vi "art联动采集V4.0.vi"() -> ()   [LabVIEW 2016]
uses:
  <vilib>/Instr/_visa.llb/VISA Configure Serial Port (Instr).vi
  <vilib>/Utility/file.llb/Write Delimited Spreadsheet (DBL).vi
panel:
  in  "定位模式":bool
  in  "X终点":dbl
  in  "Y终点":dbl
  in  "高级设置":bool
  in  "Y轴回零速度":dbl=15000.0
  in  "X轴回零速度":dbl=15000.0
  in  "细分设置":dbl=8.0
  in  "等待时间":u32=40
  in  "文件保存":path=path "D:/" caption="保存路径"
  out "行用时（s）":dbl
  out "time（行）":u32
  out "hDevice out":i32=253955776
  out "error out":errorcluster caption="错误输出"
  in  "退出扫描(Esc)":bool
  out "N_Length":i32=16384
  out "M_Length":i32
  out "hDevice":i32=241832032
  out "pulDDR2Length":u32=256
  out "总用时（s）":dbl
  out "毫秒计时值":u32=3586537
  out "数组":dbl[][](array[numeric])=[[58819.77200735986, 88200.32943600747]]
  out "强度图":dbl[][](graph)=[[58819.77200735986, 88200.32943600747]]
  out "judge":dbl
  out "Xloop":dbl
  out "幅频谱":dbl[](graph)
  out "时域谱":dbl[](graph)
  out "错误输出":errorcluster
  in  "启动":bool
  in  "开始扫描":bool
  in  "X归零":bool
  in  "Y归零":bool
  in  "Y起点":dbl
  in  "Y轴速度":dbl=9000.0
  in  "X轴速度":dbl=9000.0
  out "电机状态":bool
  in  "电机端口":refnum<visa-resource-name>="COM6"
  out "Yloop":dbl=1.0
  out "X扫描范围":dbl=150.0
  out "Y扫描范围":dbl=75.0
  out "Y序":i32
  in  "X起点":dbl
  out "Y(mm)":dbl
  out "x+y 2":dbl=3.0
  in  "Y步进":dbl=1.0
  in  "精度":dbl=0.001
  in  "电机急停":bool
  out "X（mm）":dbl
  out "x+y":dbl=1.0
  in  "X步进":dbl=1.0
  # "实时坐标"
  # "时域谱"
  # "频域谱"
  # "扫描参数"
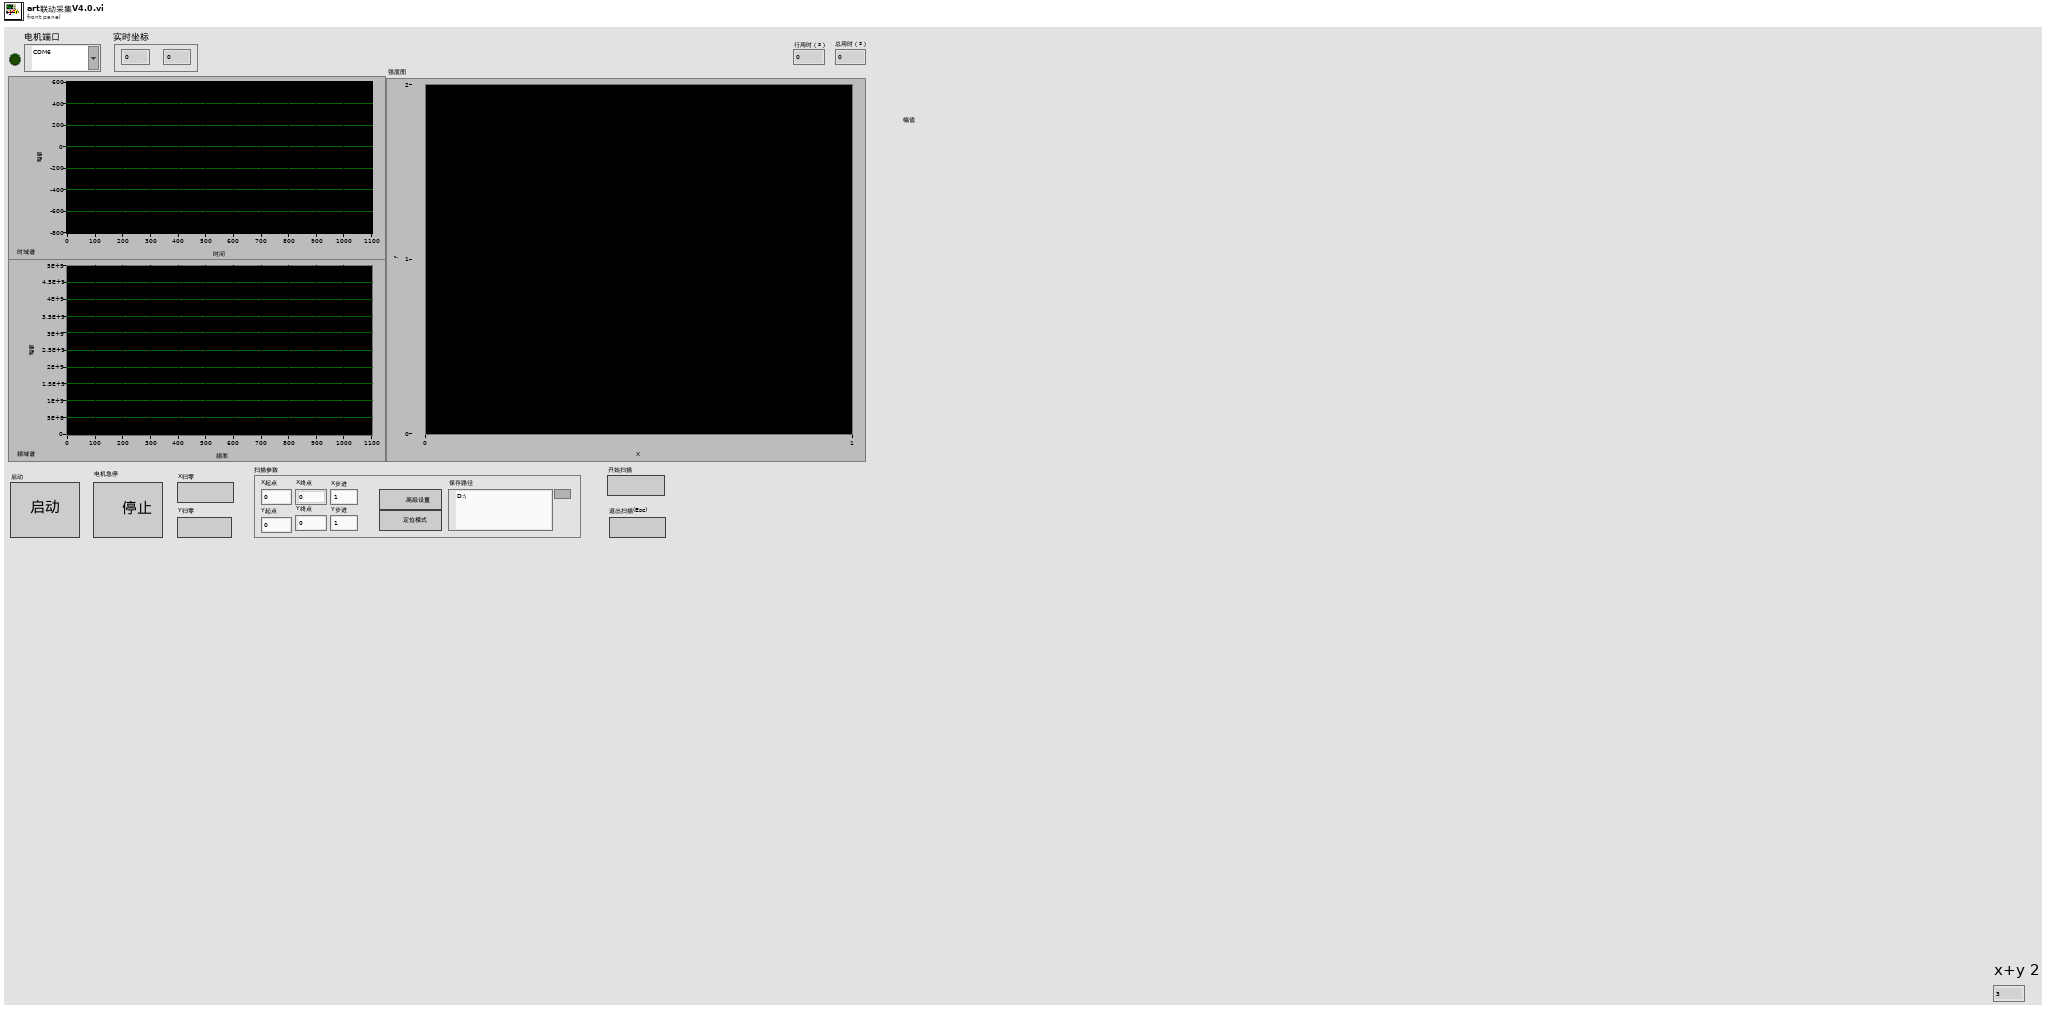
[diagram p1: front panel]
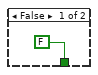
[diagram p2: hidden frame]
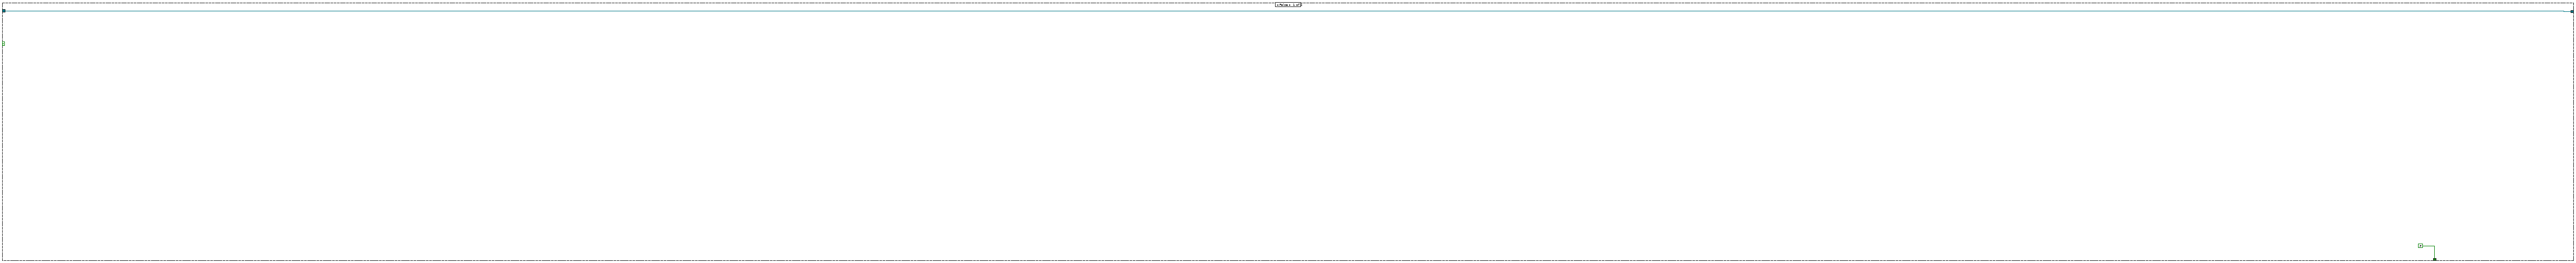
[diagram p3: hidden frame]
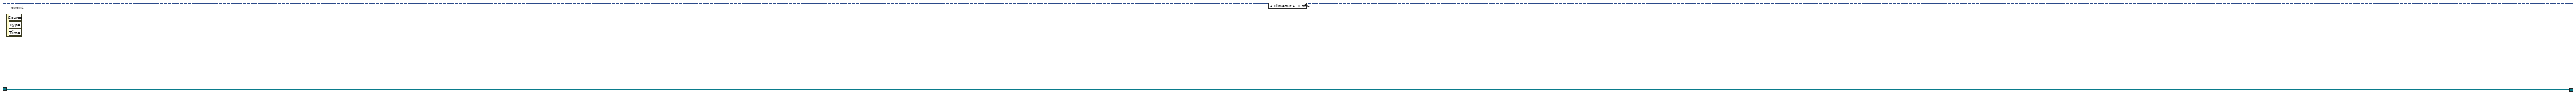
[diagram p4: hidden frame]
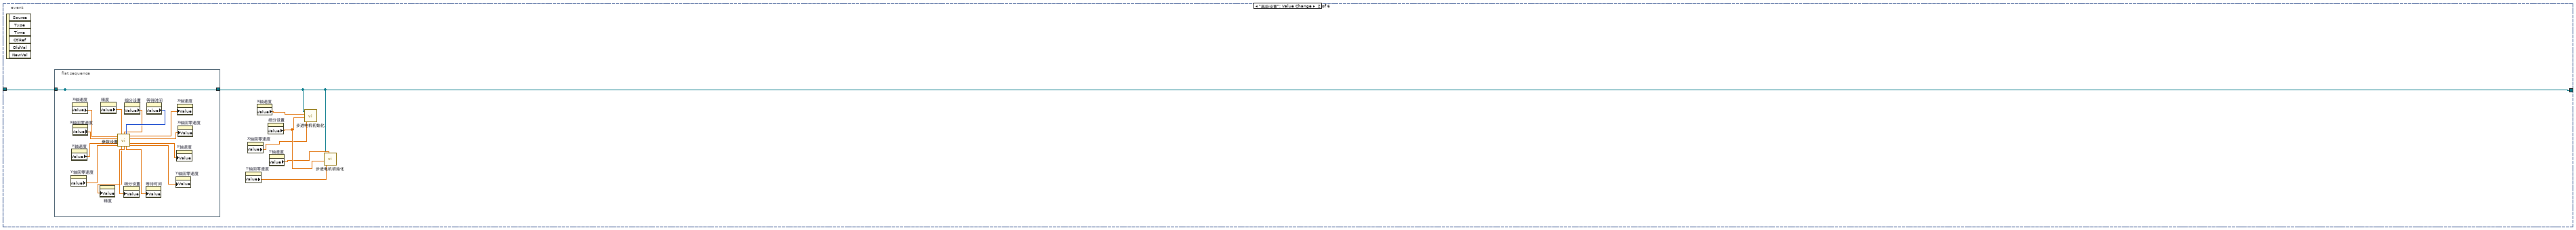
[diagram p5: hidden frame]
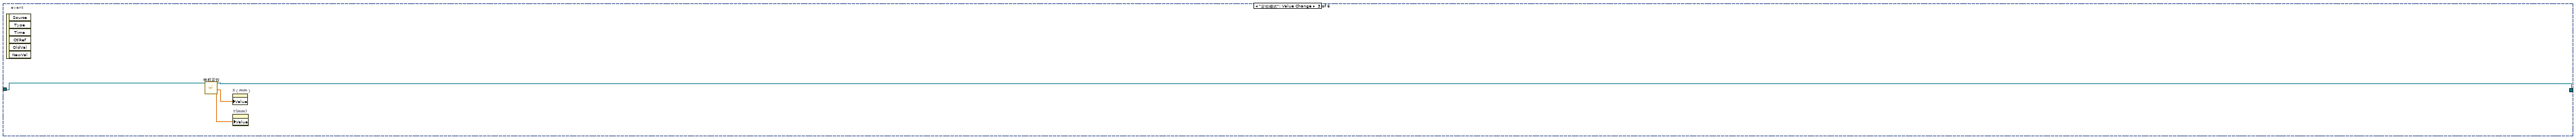
[diagram p6: hidden frame]
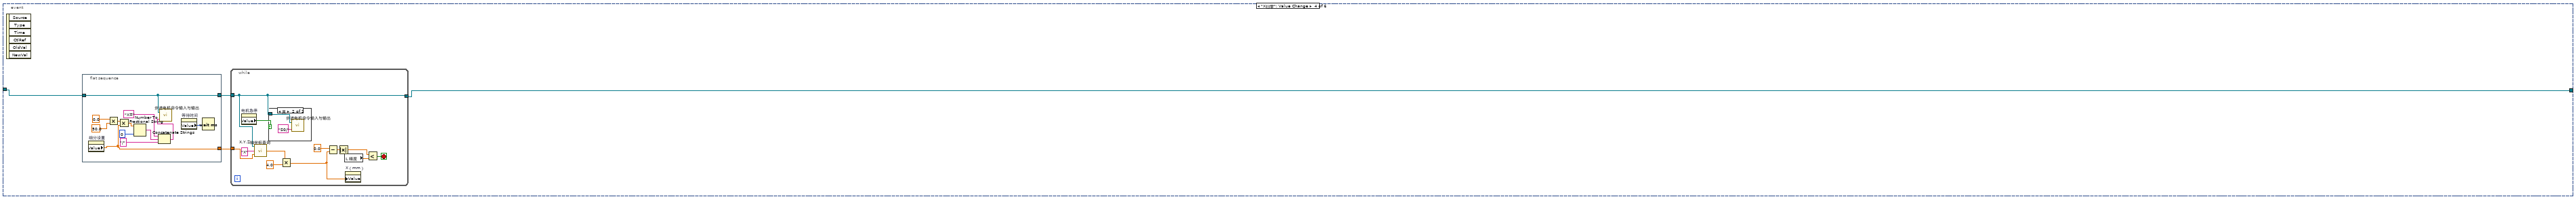
[diagram p7: hidden frame]
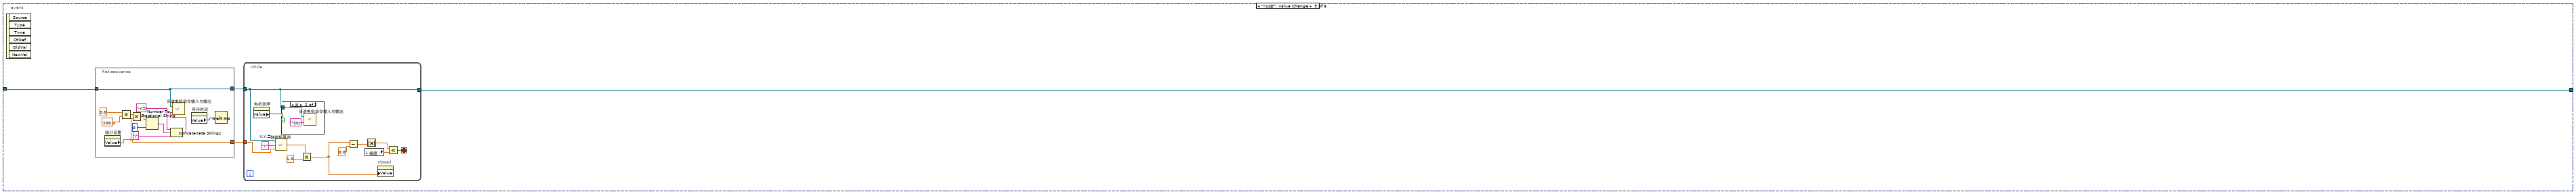
[diagram p9: hidden frame]
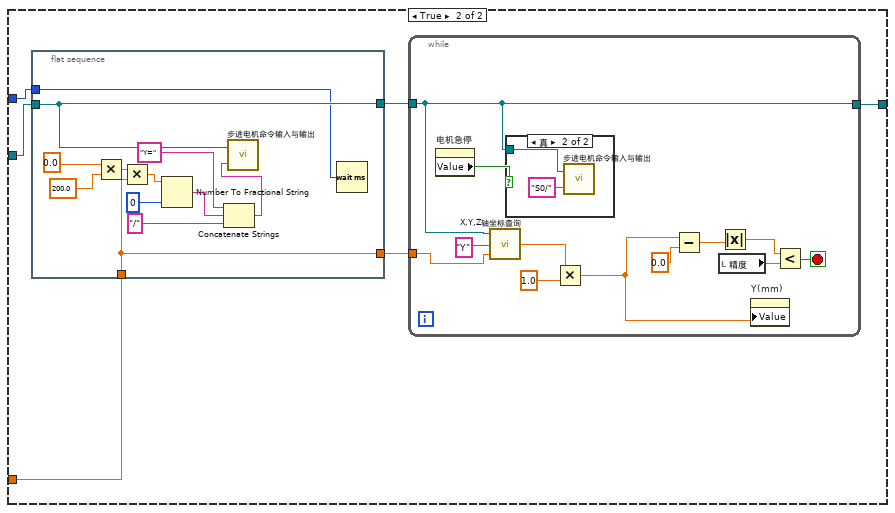
[diagram p15: hidden frame]
diagram:
  n1 = while {
    stop <- w1 stop-if-true
    n2 = case shown="真" "启动" {
      tunnel: [FALSE ("ESC") w8] -> w1
      frame False {
      }
      frame True {
        w23 = 0  # OutClockSource
        w24 = 0  # bClockSourceDir
        w26 = 10000000  # Frequency
        w27 = 0  # ClockSource
        w28 = 0  # TrigLevelVolt
        w15 = 1
        w29 = 0  # TriggerDir
        w30 = 0  # TriggerSource
        w31 = 0  # ATRTriggerChannel
        w32 = 0  # TriggerMode
        w16 = 4096  # N_Length
        w17 = 0  # M_Length
        w33 = 1  # CouplingType
        w34 = 0  # DeviceLgcID
        w44 = u16 0 items=["无", "XON/XOFF", "RTS/CTS", "XON/XOFF & RTS/CTS", "DTR/DSR", "XON/XOFF & DTR/DSR"] ("flow control (0:none)")
        w45 = u16 10 items=["1.0"=10, "1.5"=15, "2.0"=20] ("stop bits (10: 1 bit)")
        # "3"
        # "2"
        # "1"
        n3 = call-poly "VISA Configure Serial Port"("VISA resource name"="电机端口", "baud rate (9600)"=u32 9600, "data bits (8)"=u16 8, "parity (0:none)"=enum16{"None", "Odd", "Even", "Mark", "Space"}."None", "stop bits (10: 1 bit)"=w45, "flow control (0:none)"=w44) -> ("VISA resource name out"=w36:refnum<visa-resource-name>, "error out"=→"error out":errorcluster)  [unwired: 1 in, 7 out]
        n4 = Build Array "InputRange"(w15, w15, w15, w15) -> (w14:i32[])
        n5 = dll-call lib="PTH2aabs CUsersH301Desktopart闭环扫描程序采集卡控制INFamd64PCI8502_32.dll" fn="PCI8502_CreateDevice" label="CreateDevice"("DeviceLgcID"=w34) -> (w21:i32)  [unwired: 4 in, 2 out]
        n6 = property on="细分设置" class="DigNum (严格)"() -> ("Value"=w7:dbl)  [unwired: 2 in, 2 out]
        n7 = Build Array (concatenate) "InitDeviceAD"(w26, w14, w33, w17, w16, w32, w31, w30, w29, w28, w27, w24, w23) -> (w25:i32[])
        n8 = call "步进电机初始化.vi"("回零速度"="X轴回零速度", "细分设置"=w7, "X轴速度"="X轴速度", "串口通信端口"=w36) -> ()  [unwired: 2 in, 1 out]
        n9 = dll-call lib="PTH2aabs CUsersH301Desktopart闭环扫描程序采集卡控制INFamd64PCI8502_32.dll" fn="PCI8502_GetDDR2Length" label="GetDDR2Length"("hDevice"=w21, "pulDDR2Length"=u32 0) -> ("hDevice"=w20:i32, "pulDDR2Length"=→"pulDDR2Length":u32)  [unwired: 4 in, 2 out]
        n10 = call "步进电机初始化.vi"("Y轴速度"="Y轴速度", "回零速度"="Y轴回零速度", "细分设置"=w7, "串口通信端口"=w36) -> ()  [unwired: 2 in, 1 out]
        n11 = call "步进电机命令输入与输出.vi"("输入字符串"="?R/", "串口通信端口"=w36) -> ("返回字符串"=w41:string)
        n12 = dll-call lib="PTH2aabs CUsersH301Desktopart闭环扫描程序采集卡控制INFamd64PCI8502_32.dll" fn="PCI8502_InitDeviceAD" label="InitDeviceAD"("hDevice"=w20, "pADPara"=w25) -> ("hDevice"=→"hDevice":i32)  [unwired: 5 in, 2 out]
        n13 = String Subset(string=w41, offset (0)=0 ("偏移量(0)"), length (rest)=2 ("长度（剩余）")) -> (substring=w38:string)
        n14 = Equal?(x=w38, y="OK") -> (x = y?=w35:bool)
        "电机状态" <- w35
        n15 = case shown="真" w35 {
          tunnel: w36 -> [w51 w54]
          tunnel: [w51 w53] -> w9
          tunnel: [FALSE ("ESC") w52] -> w8
          frame False {
          }
          frame True {
            n16 = while {
              tunnel: w54 -> [w58]
              tunnel: [w57] -> w53
              tunnel: ["退出扫描(Esc)"] -> w52
              stop <- "退出扫描(Esc)" stop-if-true
              n17 = event shown="[5] \"开始扫描\": 值改变" {
                selector: _ -> [_ _ _ _ _ _]
                dyn-events: _ -> [_ _ _ _ _ _]
                timeout: 1 -> [_ _ _ _ _ _]
                tunnel: w58 -> [w59 w66 w85 w89 w119 w170]
                tunnel: [w59 w60 w84 w87 w117 w163] -> w57
                event Timeout {
                  n18 = event-data() -> ()  [unwired: 1 in, 3 out]
                }
                event "高级设置": Value Change {
                  n19 = event-data() -> ()  [unwired: 1 in, 6 out]
                  n20 = flat-sequence {
                    tunnel: w66 -> [w67]
                    tunnel: [w67] -> _
                    tunnel: [w67] -> w60
                    frame #0 {
                      n21 = property on="Y轴回零速度" class="DigNum (严格)"() -> ("Value"=w71:dbl)  [unwired: 2 in, 2 out]
                      n22 = property on="Y轴速度" class="DigNum (严格)"() -> ("Value"=w70:dbl)  [unwired: 2 in, 2 out]
                      n23 = property on="X轴速度" class="DigNum (严格)"() -> ("Value"=w68:dbl)  [unwired: 2 in, 2 out]
                      n24 = property on="X轴回零速度" class="DigNum (严格)"() -> ("Value"=w69:dbl)  [unwired: 2 in, 2 out]
                      n25 = property on="精度" class="DigNum (严格)"() -> ("Value"=w75:dbl)  [unwired: 2 in, 2 out]
                      n26 = property on="细分设置" class="DigNum (严格)"() -> ("Value"=w76:dbl)  [unwired: 2 in, 2 out]
                      n27 = property on="等待时间" class="DigNum (严格)"() -> ("Value"=w77:u32)  [unwired: 2 in, 2 out]
                      n28 = call "参数设置.vi"("X轴速度"=w68, "精度"=w75, "细分设置"=w76, "等待时间"=w77, "X轴回零速度"=w69, "Y轴速度"=w70, "Y轴回零速度"=w71) -> ("X轴速度"=w78:dbl, "X轴回零速度"=w79:dbl, "Y轴速度"=w80:dbl, "精度"=w72:dbl, "细分设置"=w73:dbl, "等待时间"=w74:dbl, "Y轴回零速度"=w81:dbl)  [unwired: 2 in]
                      n29 = property on="精度" class="DigNum (严格)"("Value"=w72) -> ()  [unwired: 2 in, 2 out]
                      n30 = property on="细分设置" class="DigNum (严格)"("Value"=w73) -> ()  [unwired: 2 in, 2 out]
                      n31 = property on="等待时间" class="DigNum (严格)"("Value"=w74) -> ()  [unwired: 2 in, 2 out]
                      n32 = property on="Y轴回零速度" class="DigNum (严格)"("Value"=w81) -> ()  [unwired: 2 in, 2 out]
                      n33 = property on="Y轴速度" class="DigNum (严格)"("Value"=w80) -> ()  [unwired: 2 in, 2 out]
                      n34 = property on="X轴速度" class="DigNum (严格)"("Value"=w78) -> ()  [unwired: 2 in, 2 out]
                      n35 = property on="X轴回零速度" class="DigNum (严格)"("Value"=w79) -> ()  [unwired: 2 in, 2 out]
                    }
                  }
                  n36 = property on="Y轴回零速度" class="DigNum (严格)"() -> ("Value"=w62:dbl)  [unwired: 2 in, 2 out]
                  n37 = property on="X轴回零速度" class="DigNum (严格)"() -> ("Value"=w63:dbl)  [unwired: 2 in, 2 out]
                  n38 = property on="X轴速度" class="DigNum (严格)"() -> ("Value"=w64:dbl)  [unwired: 2 in, 2 out]
                  n39 = property on="细分设置" class="DigNum (严格)"() -> ("Value"=w65:dbl)  [unwired: 2 in, 2 out]
                  n40 = property on="Y轴速度" class="DigNum (严格)"() -> ("Value"=w61:dbl)  [unwired: 2 in, 2 out]
                  n41 = call "步进电机初始化.vi"("回零速度"=w63, "细分设置"=w65, "X轴速度"=w64, "串口通信端口"=w60) -> ()  [unwired: 2 in, 1 out]
                  n42 = call "步进电机初始化.vi"("Y轴速度"=w61, "回零速度"=w62, "细分设置"=w65, "串口通信端口"=w60) -> ()  [unwired: 2 in, 1 out]
                }
                event "定位模式": Value Change {
                  n43 = event-data() -> ()  [unwired: 1 in, 6 out]
                  n44 = call "电机定位.vi"("VISA I"=w85) -> ("Y"=w82:dbl, "X"=w83:dbl, "VISA O"=w84:refnum<visa-resource-name>)  [unwired: 8 in]
                  n45 = property on="X（mm）" class="DigNum (严格)"("Value"=w83) -> ()  [unwired: 2 in, 2 out]
                  n46 = property on="Y(mm)" class="DigNum (严格)"("Value"=w82) -> ()  [unwired: 2 in, 2 out]
                }
                event "X归零": Value Change {
                  n47 = event-data() -> ()  [unwired: 1 in, 6 out]
                  n48 = flat-sequence {
                    tunnel: w89 -> [w93]
                    tunnel: [w93] -> w88
                    tunnel: [w90] -> w86
                    frame #0 {
                      n49 = property on="细分设置" class="DigNum (严格)"() -> ("Value"=w90:dbl)  [unwired: 2 in, 2 out]
                      n50 = Multiply(x=0.0, y=50.0) -> (x*y=w96:dbl)
                      n51 = Multiply(x=w96, y=w90) -> (x*y=w101:dbl)
                      n52 = Number To Fractional String(number=w101, precision (6)=i16 0 ("精度(6)")) -> (F-format string=w99:string)  [unwired: 2 out]
                      n53 = Concatenate Strings("X=" ("字符串"), w99, "/" ("字符串")) -> (w94:string)
                      n54 = call "步进电机命令输入与输出.vi"("输入字符串"=w94, "串口通信端口"=w93) -> ()  [unwired: 1 out]
                      n55 = property on="等待时间" class="DigNum (严格)"() -> ("Value"=w91:u32)  [unwired: 2 in, 2 out]
                      n56 = Wait (ms)(milliseconds to wait=w91) -> ()  [unwired: 1 out]
                    }
                  }
                  n57 = while {
                    tunnel: [w103] -> w87
                    tunnel: w88 -> [w103]
                    tunnel: w86 -> [w102]
                    stop <- w109 stop-if-true
                    n58 = property on="电机急停" class="Bool (严格)"() -> ("Value"=w110:bool)  [unwired: 2 in, 2 out]
                    n59 = call "X,Y,Z轴坐标查询.vi"("细分设置"=w102, "查询坐标轴"="X", "串口通信端口"=w103) -> ("坐标(mm)"=w111:dbl)
                    n60 = case shown="真" w110 {
                      tunnel: w103 -> [_ w114]
                      frame False {
                      }
                      frame True {
                        n61 = call "步进电机命令输入与输出.vi"("输入字符串"="S0/", "串口通信端口"=w114) -> ()  [unwired: 1 out]
                      }
                    }
                    n62 = Multiply(x=w111, y=4.0 ("x")) -> (x*y=w107:dbl)
                    n63 = Subtract(x=0.0, y=w107) -> (x-y=w106:dbl)
                    n64 = Absolute Value(x=w106) -> (abs(x)=w105:dbl)
                    n65 = local read "精度"() -> (w108:dbl)
                    n66 = property on="X（mm）" class="DigNum (严格)"("Value"=w107) -> ()  [unwired: 2 in, 2 out]
                    n67 = Less?(x=w105, y=w108) -> (x < y?=w109:bool)
                  }
                }
                event "Y归零": Value Change {
                  n68 = event-data() -> ()  [unwired: 1 in, 6 out]
                  n69 = flat-sequence {
                    tunnel: w119 -> [w123]
                    tunnel: [w123] -> w118
                    tunnel: [w120] -> w116
                    frame #0 {
                      n70 = property on="细分设置" class="DigNum (严格)"() -> ("Value"=w120:dbl)  [unwired: 2 in, 2 out]
                      n71 = Multiply(x=0.0, y=200.0) -> (x*y=w126:dbl)
                      n72 = Multiply(x=w126, y=w120) -> (x*y=w131:dbl)
                      n73 = Number To Fractional String(number=w131, precision (6)=i16 0 ("精度(6)")) -> (F-format string=w129:string)  [unwired: 2 out]
                      n74 = Concatenate Strings("Y=" ("字符串"), w129, "/" ("字符串")) -> (w124:string)
                      n75 = call "步进电机命令输入与输出.vi"("输入字符串"=w124, "串口通信端口"=w123) -> ()  [unwired: 1 out]
                      n76 = property on="等待时间" class="DigNum (严格)"() -> ("Value"=w121:u32)  [unwired: 2 in, 2 out]
                      n77 = Wait (ms)(milliseconds to wait=w121) -> ()  [unwired: 1 out]
                    }
                  }
                  n78 = while {
                    tunnel: [w133] -> w117
                    tunnel: w118 -> [w133]
                    tunnel: w116 -> [w132]
                    stop <- w139 stop-if-true
                    n79 = property on="电机急停" class="Bool (严格)"() -> ("Value"=w140:bool)  [unwired: 2 in, 2 out]
                    n80 = call "X,Y,Z轴坐标查询.vi"("细分设置"=w132, "查询坐标轴"="Y", "串口通信端口"=w133) -> ("坐标(mm)"=w141:dbl)
                    n81 = case shown="真" w140 {
                      tunnel: w133 -> [_ w144]
                      frame False {
                      }
                      frame True {
                        n82 = call "步进电机命令输入与输出.vi"("输入字符串"="S0/", "串口通信端口"=w144) -> ()  [unwired: 1 out]
                      }
                    }
                    n83 = Multiply(x=w141, y=1.0 ("x")) -> (x*y=w137:dbl)
                    n84 = Subtract(x=w137, y=0.0 ("x")) -> (x-y=w135:dbl)
                    n85 = local read "精度"() -> (w138:dbl)
                    n86 = Absolute Value(x=w135) -> (abs(x)=w134:dbl)
                    n87 = property on="Y(mm)" class="DigNum (严格)"("Value"=w137) -> ()  [unwired: 2 in, 2 out]
                    n88 = Less?(x=w134, y=w138) -> (x < y?=w139:bool)
                  }
                }
                event "开始扫描": Value Change {
                  n89 = event-data() -> ()  [unwired: 1 in, 6 out]
                  n90 = flat-sequence {
                    tunnel: w170 -> [w187]
                    tunnel: [w187] -> w159
                    frame #0 {
                      # "如果强度图那里出了错，就把这里的行列互换"
                      n91 = local read "Xloop"() -> (w182:dbl)
                      n92 = local read "Yloop"() -> (w181:dbl)
                      n93 = Multiply(x="Y起点", y=200.0) -> (x*y=w190:dbl)
                      n94 = Tick Count (ms)() -> (millisecond timer value=→"毫秒计时值":u32)
                      n95 = Multiply(x=w190, y="细分设置") -> (x*y=w195:dbl)
                      n96 = Initialize Array(0.0 ("元素"), w182, w181) -> (→"强度图":dbl[][])
                      n97 = Number To Fractional String(number=w195, precision (6)=i16 0 ("精度(6)")) -> (F-format string=w193:string)  [unwired: 2 out]
                      n98 = Concatenate Strings("Y=" ("字符串"), w193, "/" ("字符串")) -> (w188:string)
                      n99 = call "步进电机命令输入与输出.vi"("输入字符串"=w188, "串口通信端口"=w187) -> ()  [unwired: 1 out]
                      n100 = property on="等待时间" class="DigNum (严格)"() -> ("Value"=w179:u32)  [unwired: 2 in, 2 out]
                      n101 = Wait (ms)(milliseconds to wait=w179) -> ()  [unwired: 1 out]
                    }
                  }
                  n102 = local read "X起点"() -> (w155:dbl)
                  n103 = Subtract(x="X终点", y=w155) -> (x-y=w154:dbl)
                  "X扫描范围" <- w154
                  n104 = local read "X步进"() -> (w162:dbl)
                  n105 = Divide(x=w154, y=w162) -> (x/y=w160:dbl)
                  n106 = Increment(x=w160) -> (x+1=→"Xloop":dbl)
                  n107 = while {
                    tunnel: [w196] -> w169
                    tunnel: w159 -> [w196]
                    stop <- w201 stop-if-true
                    n108 = call "X,Y,Z轴坐标查询.vi"("细分设置"=8.0, "查询坐标轴"="Y", "串口通信端口"=w196) -> ("坐标(mm)"=w203:dbl)
                    n109 = property on="Y起点" class="DigNum (严格)"() -> ("Value"=w205:dbl)  [unwired: 2 in, 2 out]
                    n110 = property on="电机急停" class="Bool (严格)"() -> ("Value"=w202:bool)  [unwired: 2 in, 2 out]
                    n111 = Multiply(x=w203, y=1.0 ("x")) -> (x*y=w199:dbl)
                    n112 = Subtract(x=w205, y=w199) -> (x-y=w198:dbl)
                    n113 = case shown="真" w202 {
                      tunnel: w196 -> [_ w208]
                      frame False {
                      }
                      frame True {
                        n114 = call "步进电机命令输入与输出.vi"("输入字符串"="S0/", "串口通信端口"=w208) -> ()  [unwired: 1 out]
                      }
                    }
                    n115 = Absolute Value(x=w198) -> (abs(x)=w197:dbl)
                    n116 = local read "精度"() -> (w200:dbl)
                    n117 = property on="Y(mm)" class="DigNum (严格)"("Value"=w199) -> ()  [unwired: 2 in, 2 out]
                    n118 = Less?(x=w197, y=w200) -> (x < y?=w201:bool)
                  }
                  n119 = local read "Y起点"() -> (w157:dbl)
                  n120 = local read "Y步进"() -> (w168:dbl)
                  n121 = Subtract(x="Y终点", y=w157) -> (x-y=w153:dbl)
                  "Y扫描范围" <- w153
                  n122 = Divide(x=w153, y=w168) -> (x/y=w167:dbl)
                  n123 = Increment(x=w167) -> (x+1=w166:dbl)
                  "Yloop" <- w166
                  n124 = Build Path(base path="文件保存", name or relative path="频域谱" ("名称或相对路径")) -> (appended path=w150:path)
                  n125 = Create Folder(path (use dialog)=w150) -> (created path=w146:path)  [unwired: 2 in, 2 out]
                  n126 = Build Path(base path="文件保存", name or relative path="时域谱" ("名称或相对路径")) -> (appended path=w152:path)
                  n127 = Create Folder(path (use dialog)=w152) -> (created path=w147:path)  [unwired: 2 in, 2 out]
                  n128 = for {
                    N: w166 -> [_]
                    tunnel: w169 -> [w229]
                    shift-right: [w228] -> w165
                    shift-left: _ -> [_]
                    tunnel: [w222] -> w164 mode=indexing
                    tunnel: w147 -> [w211]
                    tunnel: w146 -> [w210]
                    i -> [w230]
                    n129 = flat-sequence {
                      tunnel: w229 -> [w288]
                      tunnel: [w288] -> w227
                      tunnel: [w284] -> w215
                      frame #0 {
                        n130 = property on="细分设置" class="DigNum (严格)"() -> ("Value"=w284:dbl)  [unwired: 2 in, 2 out]
                        n131 = Multiply(x="X起点", y=50.0) -> (x*y=w291:dbl)
                        n132 = Multiply(x=w291, y=w284) -> (x*y=w296:dbl)
                        n133 = Number To Fractional String(number=w296, precision (6)=i16 0 ("精度(6)")) -> (F-format string=w294:string)  [unwired: 2 out]
                        n134 = Concatenate Strings("X=" ("字符串"), w294, "/" ("字符串")) -> (w289:string)
                        n135 = call "步进电机命令输入与输出.vi"("输入字符串"=w289, "串口通信端口"=w288) -> ()  [unwired: 1 out]
                        n136 = Tick Count (ms)() -> (millisecond timer value=→"time（行）":u32)
                        n137 = Wait (ms)(milliseconds to wait="等待时间") -> ()  [unwired: 1 out]
                      }
                    }
                    n138 = while {
                      tunnel: [w298] -> w231
                      tunnel: w227 -> [w298]
                      tunnel: w215 -> [w297]
                      stop <- w303 stop-if-true
                      n139 = property on="电机急停" class="Bool (严格)"() -> ("Value"=w304:bool)  [unwired: 2 in, 2 out]
                      n140 = case shown="真" w304 {
                        tunnel: w298 -> [_ w309]
                        frame False {
                        }
                        frame True {
                          n141 = call "步进电机命令输入与输出.vi"("输入字符串"="S0/", "串口通信端口"=w309) -> ()  [unwired: 1 out]
                        }
                      }
                      n142 = call "X,Y,Z轴坐标查询.vi"("细分设置"=w297, "查询坐标轴"="X", "串口通信端口"=w298) -> ("坐标(mm)"=w305:dbl)
                      n143 = Multiply(x=w305, y=4.0 ("x")) -> (x*y=w301:dbl)
                      n144 = property on="X起点" class="DigNum (严格)"() -> ("Value"=w307:dbl)  [unwired: 2 in, 2 out]
                      n145 = Subtract(x=w307, y=w301) -> (x-y=w300:dbl)
                      n146 = Absolute Value(x=w300) -> (abs(x)=w299:dbl)
                      n147 = local read "精度"() -> (w302:dbl)
                      n148 = property on="X（mm）" class="DigNum (严格)"("Value"=w301) -> ()  [unwired: 2 in, 2 out]
                      n149 = Less?(x=w299, y=w302) -> (x < y?=w303:bool)
                    }
                    n150 = local read "Xloop"() -> (w216:dbl)
                    n151 = for {
                      N: w216 -> [_]
                      tunnel: w231 -> [w383]
                      shift-right: [w381] -> w224
                      shift-left: _ -> [_]
                      tunnel: [w380] -> w226 mode=indexing
                      tunnel: [w379] -> w225 mode=indexing
                      tunnel: [w378] -> w222 mode=indexing
                      i -> [w377]
                      n152 = flat-sequence {
                        tunnel: w383 -> [w387]
                        tunnel: [w386] -> w382
                        tunnel: w377 -> [w384]
                        tunnel: [w437] -> w381
                        tunnel: w382 -> [w437]
                        tunnel: [w436] -> w380
                        tunnel: [w435] -> w379
                        tunnel: [w431] -> w378
                        frame #0 {
                          n153 = Equal To 0?(x=w384) -> (x = 0?=w385:bool)
                          n154 = case shown="假" w385 {
                            tunnel: w387 -> [w390 w425]
                            tunnel: [w389 w425] -> w386
                            frame False {
                              n155 = flat-sequence {
                                tunnel: w390 -> [w400]
                                tunnel: [w400] -> w391
                                tunnel: [w392] -> w388
                                frame #0 {
                                n156 = local read "X步进"() -> (w394:dbl)
                                n157 = Multiply(x=w394, y=1.0 ("x")) -> (x*y=w399:dbl)
                                n158 = property on="等待时间" class="DigNum (严格)"() -> ("Value"=w393:u32)  [unwired: 2 in, 2 out]
                                n159 = property on="细分设置" class="DigNum (严格)"() -> ("Value"=w392:dbl)  [unwired: 2 in, 2 out]
                                n160 = call "X,Y,Z轴坐标查询.vi"("细分设置"=w392, "查询坐标轴"="X", "串口通信端口"=w400) -> ("坐标(mm)"=w396:dbl)
                                n161 = Multiply(x=4.0, y=w396) -> (x*y=w395:dbl)
                                n162 = Add(x=w395, y=w399) -> (x+y=w402:dbl)
                                "x+y" <- w402
                                n163 = Multiply(x=w402, y=50.0) -> (x*y=w405:dbl)
                                n164 = Multiply(x=w405, y=w392) -> (x*y=w410:dbl)
                                n165 = Number To Fractional String(number=w410, precision (6)=i16 0 ("精度(6)")) -> (F-format string=w408:string)  [unwired: 2 out]
                                n166 = Concatenate Strings("X=" ("字符串"), w408, "/" ("字符串")) -> (w403:string)
                                n167 = call "步进电机命令输入与输出.vi"("输入字符串"=w403, "串口通信端口"=w400) -> ()  [unwired: 1 out]
                                n168 = Wait (ms)(milliseconds to wait=w393) -> ()  [unwired: 1 out]
                                }
                              }
                              n169 = while {
                                tunnel: [w420] -> w389
                                tunnel: w391 -> [w420]
                                tunnel: w388 -> [w411]
                                stop <- w419 stop-if-true
                                n170 = property on="电机急停" class="Bool (严格)"() -> ("Value"=w417:bool)  [unwired: 2 in, 2 out]
                                n171 = local read "x+y"() -> (w421:dbl)
                                n172 = case shown="真" w417 {
                                tunnel: w420 -> [_ w423]
                                frame False {
                                }
                                frame True {
                                n173 = call "步进电机命令输入与输出.vi"("输入字符串"="S0/", "串口通信端口"=w423) -> ()  [unwired: 1 out]
                                }
                                }
                                n174 = call "X,Y,Z轴坐标查询.vi"("细分设置"=w411, "查询坐标轴"="X", "串口通信端口"=w420) -> ("坐标(mm)"=w415:dbl)
                                n175 = Multiply(x=4.0, y=w415) -> (x*y=w414:dbl)
                                n176 = Subtract(x=w421, y=w414) -> (x-y=w413:dbl)
                                n177 = property on="X（mm）" class="DigNum (严格)"("Value"=w414) -> ()  [unwired: 2 in, 2 out]
                                n178 = Absolute Value(x=w413) -> (abs(x)=w412:dbl)
                                n179 = local read "精度"() -> (w416:dbl)
                                n180 = Less?(x=w412, y=w416) -> (x < y?=w419:bool)
                              }
                            }
                            frame True {
                            }
                          }
                        }
                        frame #1 {
                          n181 = local read "pulDDR2Length"() -> (w430:u32)
                          n182 = local read "hDevice"() -> (w429:i32)
                          n183 = local read "M_Length"() -> (w428:i32)
                          n184 = local read "N_Length"() -> (w427:i32)
                          n185 = call "AD（V3.1）.vi"("N-length"=w427, "M-length"=w428, "hDevice"=w429, "pulDDR2Length"=w430) -> ("幅频谱"=w435:dbl[], "时域谱"=w436:dbl[], "hDevice out"=→"hDevice out":i32)  [unwired: 5 in]
                          "时域谱" <- w436
                          "幅频谱" <- w435
                          n186 = Array Subset(array=w435, index=60 ("索引"), length=453 ("长度")) -> (w432:dbl[])
                          n187 = Array Max & Min(array=w432) -> (max value=w431:dbl)  [unwired: 3 out]
                        }
                      }
                    }
                    n188 = flat-sequence {
                      tunnel: w225 -> [w265]
                      tunnel: w226 -> [w273]
                      tunnel: w224 -> [w282]
                      tunnel: [w282] -> w218
                      tunnel: w211 -> [w260]
                      tunnel: w210 -> [w259]
                      frame #0 {
                        n189 = local read "time（行）"() -> (w281:u32)
                        n190 = Tick Count (ms)() -> (millisecond timer value=w277:u32)
                        n191 = Subtract(x=w277, y=w281) -> (x-y=w280:u32)
                        n192 = local read "Y序"() -> (w261:i32)
                        n193 = Multiply(x=w280, y=0.001) -> (x*y=→"行用时（s）":dbl)
                        n194 = Increment(x=w261) -> (x+1=w262:i32)
                        n195 = Number To Decimal String(number=w262) -> (decimal integer string=w271:string)  [unwired: 1 in]
                        n196 = Number To Decimal String(number=w262) -> (decimal integer string=w270:string)  [unwired: 1 in]
                        n197 = Concatenate Strings("T" ("字符串"), w271, ".txt" ("字符串")) -> (w274:string)
                        n198 = Concatenate Strings("F" ("字符串"), w270, ".txt" ("字符串")) -> (w268:string)
                        n199 = Build Path(base path=w260, name or relative path=w274) -> (appended path=w276:path)
                        n200 = call-poly <vilib>:"Write Delimited Spreadsheet.vi"("file path (dialog if empty)"=w276, "2D data"=w273, "transpose? (no:F)"=FALSE) -> ()  [unwired: 11 in, 2 out]
                        n201 = Build Path(base path=w259, name or relative path=w268) -> (appended path=w266:path)
                        n202 = call-poly <vilib>:"Write Delimited Spreadsheet.vi"("file path (dialog if empty)"=w266, "2D data"=w265, "transpose? (no:F)"=FALSE) -> ()  [unwired: 11 in, 2 out]
                        "judge" <- 1.0
                      }
                    }
                    n203 = flat-sequence {
                      tunnel: w218 -> [w236]
                      tunnel: [w236] -> w219
                      tunnel: [w234] -> w214
                      frame #0 {
                        n204 = property on="细分设置" class="DigNum (严格)"() -> ("Value"=w234:dbl)  [unwired: 2 in, 2 out]
                        n205 = property on="等待时间" class="DigNum (严格)"() -> ("Value"=w233:u32)  [unwired: 2 in, 2 out]
                        n206 = Multiply(x=0.0, y=50.0) -> (x*y=w239:dbl)
                        n207 = Multiply(x=w239, y=w234) -> (x*y=w244:dbl)
                        n208 = Wait (ms)(milliseconds to wait=w233) -> ()  [unwired: 1 out]
                        n209 = Number To Fractional String(number=w244, precision (6)=i16 0 ("精度(6)")) -> (F-format string=w242:string)  [unwired: 2 out]
                        n210 = Concatenate Strings("X=" ("字符串"), w242, "/" ("字符串")) -> (w237:string)
                        n211 = call "步进电机命令输入与输出.vi"("输入字符串"=w237, "串口通信端口"=w236) -> ()  [unwired: 1 out]
                      }
                    }
                    n212 = while {
                      tunnel: [w246] -> w217
                      tunnel: w219 -> [w246]
                      tunnel: w214 -> [w245]
                      stop <- w252 stop-if-true
                      n213 = property on="电机急停" class="Bool (严格)"() -> ("Value"=w253:bool)  [unwired: 2 in, 2 out]
                      n214 = call "X,Y,Z轴坐标查询.vi"("细分设置"=w245, "查询坐标轴"="X", "串口通信端口"=w246) -> ("坐标(mm)"=w254:dbl)
                      n215 = case shown="真" w253 {
                        tunnel: w246 -> [_ w257]
                        frame False {
                        }
                        frame True {
                          n216 = call "步进电机命令输入与输出.vi"("输入字符串"="S0/", "串口通信端口"=w257) -> ()  [unwired: 1 out]
                        }
                      }
                      n217 = Multiply(x=w254, y=4.0 ("x")) -> (x*y=w250:dbl)
                      n218 = Subtract(x=0.0, y=w250) -> (x-y=w249:dbl)
                      n219 = Absolute Value(x=w249) -> (abs(x)=w248:dbl)
                      n220 = local read "精度"() -> (w251:dbl)
                      n221 = property on="X（mm）" class="DigNum (严格)"("Value"=w250) -> ()  [unwired: 2 in, 2 out]
                      n222 = Less?(x=w248, y=w251) -> (x < y?=w252:bool)
                    }
                    n223 = local read "Yloop"() -> (w220:dbl)
                    n224 = Decrement(x=w220) -> (x-1=w221:dbl)
                    n225 = local read "Y序"() -> (w223:i32)
                    n226 = Equal?(x=w223, y=w221) -> (x = y?=w232:bool)
                    n227 = Increment(x=w223) -> ()  [unwired: 1 out]
                    n228 = property on="细分设置" class="DigNum (严格)"() -> ("Value"=w212:dbl)  [unwired: 2 in, 2 out]
                    n229 = property on="等待时间" class="DigNum (严格)"() -> ("Value"=w213:u32)  [unwired: 2 in, 2 out]
                    n230 = case shown="假" w232 {
                      tunnel: w217 -> [w316 w348]
                      tunnel: [w314 w349] -> w228
                      tunnel: w213 -> [w312 w346]
                      tunnel: w212 -> [w311 w345]
                      frame False {
                        n231 = flat-sequence {
                          tunnel: w316 -> [w319]
                          tunnel: [w319] -> w315
                          tunnel: [w317] -> w313
                          tunnel: w312 -> [w318]
                          tunnel: w311 -> [w317]
                          frame #0 {
                            n232 = call "X,Y,Z轴坐标查询.vi"("细分设置"=w317, "查询坐标轴"="Y", "串口通信端口"=w319) -> ("坐标(mm)"=w321:dbl)
                            n233 = local read "Y步进"() -> (w320:dbl)
                            n234 = Add(x=w321, y=w320) -> (x+y=w323:dbl)
                            "x+y 2" <- w323
                            n235 = Multiply(x=w323, y=200.0) -> (x*y=w327:dbl)
                            n236 = Multiply(x=w327, y=8.0 ("细分设置")) -> (x*y=w332:dbl)
                            n237 = Number To Fractional String(number=w332, precision (6)=i16 0 ("精度(6)")) -> (F-format string=w330:string)  [unwired: 2 out]
                            n238 = Concatenate Strings("Y=" ("字符串"), w330, "/" ("字符串")) -> (w325:string)
                            n239 = call "步进电机命令输入与输出.vi"("输入字符串"=w325, "串口通信端口"=w319) -> ()  [unwired: 1 out]
                            n240 = Wait (ms)(milliseconds to wait=w318) -> ()  [unwired: 1 out]
                          }
                        }
                        n241 = while {
                          tunnel: [w334] -> w314
                          tunnel: w315 -> [w334]
                          tunnel: w313 -> [w333]
                          stop <- w340 stop-if-true
                          n242 = call "X,Y,Z轴坐标查询.vi"("细分设置"=w333, "查询坐标轴"="Y", "串口通信端口"=w334) -> ("坐标(mm)"=w338:dbl)
                          n243 = local read "x+y 2"() -> (w341:dbl)
                          n244 = property on="电机急停" class="Bool (严格)"() -> ("Value"=w337:bool)  [unwired: 2 in, 2 out]
                          n245 = property on="Y(mm)" class="DigNum (严格)"("Value"=w338) -> ()  [unwired: 2 in, 2 out]
                          n246 = case shown="真" w337 {
                            tunnel: w334 -> [_ w343]
                            frame False {
                            }
                            frame True {
                              n247 = call "步进电机命令输入与输出.vi"("输入字符串"="S0/", "串口通信端口"=w343) -> ()  [unwired: 1 out]
                            }
                          }
                          n248 = Subtract(x=w341, y=w338) -> (x-y=w336:dbl)
                          n249 = Absolute Value(x=w336) -> (abs(x)=w335:dbl)
                          n250 = local read "精度"() -> (w339:dbl)
                          n251 = Less?(x=w335, y=w339) -> (x < y?=w340:bool)
                        }
                      }
                      frame True {
                        n252 = flat-sequence {
                          tunnel: [w353] -> _
                          tunnel: [w353] -> w350
                          tunnel: w348 -> [w353]
                          tunnel: [w351] -> w347
                          tunnel: w346 -> [w352]
                          tunnel: w345 -> [w351]
                          frame #0 {
                            n253 = Multiply(x=0.0, y=200.0) -> (x*y=w357:dbl)
                            n254 = Multiply(x=w357, y=w351) -> (x*y=w362:dbl)
                            n255 = Number To Fractional String(number=w362, precision (6)=i16 0 ("精度(6)")) -> (F-format string=w360:string)  [unwired: 2 out]
                            n256 = Concatenate Strings("Y=" ("字符串"), w360, "/" ("字符串")) -> (w355:string)
                            n257 = call "步进电机命令输入与输出.vi"("输入字符串"=w355, "串口通信端口"=w353) -> ()  [unwired: 1 out]
                            n258 = Wait (ms)(milliseconds to wait=w352) -> ()  [unwired: 1 out]
                          }
                        }
                        n259 = while {
                          tunnel: [w364] -> w349
                          tunnel: w350 -> [w364]
                          tunnel: w347 -> [w363]
                          stop <- w370 stop-if-true
                          n260 = property on="电机急停" class="Bool (严格)"() -> ("Value"=w371:bool)  [unwired: 2 in, 2 out]
                          n261 = call "X,Y,Z轴坐标查询.vi"("细分设置"=w363, "查询坐标轴"="Y", "串口通信端口"=w364) -> ("坐标(mm)"=w372:dbl)
                          n262 = case shown="真" w371 {
                            tunnel: w364 -> [_ w375]
                            frame False {
                            }
                            frame True {
                              n263 = call "步进电机命令输入与输出.vi"("输入字符串"="S0/", "串口通信端口"=w375) -> ()  [unwired: 1 out]
                            }
                          }
                          n264 = Multiply(x=w372, y=1.0 ("x")) -> (x*y=w368:dbl)
                          n265 = Subtract(x=w368, y=0.0 ("x")) -> (x-y=w366:dbl)
                          n266 = local read "精度"() -> (w369:dbl)
                          n267 = Absolute Value(x=w366) -> (abs(x)=w365:dbl)
                          n268 = property on="Y(mm)" class="DigNum (严格)"("Value"=w368) -> ()  [unwired: 2 in, 2 out]
                          n269 = Less?(x=w365, y=w369) -> (x < y?=w370:bool)
                        }
                      }
                    }
                    "Y序" <- w230
                  }
                  n270 = flat-sequence {
                    tunnel: w165 -> [w173]
                    tunnel: w164 -> [w172]
                    tunnel: [w173] -> w163
                    frame #0 {
                      n271 = local read "毫秒计时值"() -> (w177:u32)
                      n272 = Transpose 2D Array(2D array=w172) -> (transposed array=w171:dbl[][])
                      n273 = Tick Count (ms)() -> (millisecond timer value=w178:u32)
                      n274 = property on="强度图" class="IntGraph (严格)"("Value"=w171) -> ()  [unwired: 2 in, 2 out]
                      n275 = Subtract(x=w178, y=w177) -> (x-y=w174:u32)
                      n276 = Multiply(x=w174, y=0.001) -> (x*y=→"总用时（s）":dbl)
                      "数组" <- w172
                    }
                  }
                }
              }
            }
          }
        }
        n277 = local read "hDevice out"() -> (w12:i32)
        n278 = dll-call lib="PTH2]abs CUsersH301Desktopart闭环扫描程序采集卡控制INFamd64\nPCI8502_32" fn="PCI8502_ReleaseDeviceAD" label="ReleaseDeviceAD"("hDevice"=w12) -> ("hDevice"=w11:i32)  [unwired: 4 in, 2 out]
        n279 = VISA Close(VISA resource name=w9) -> (error out=→"错误输出":errorcluster)  [unwired: 1 in]
        n280 = dll-call lib="PTH2]abs CUsersH301Desktopart闭环扫描程序采集卡控制INFamd64\nPCI8502_32" fn="PCI8502_ReleaseDevice" label="ReleaseDevice"("hDevice"=w11) -> ()  [unwired: 5 in, 2 out]
        "M_Length" <- w17
        "N_Length" <- w16
      }
    }
  }
